vi "Add.vi"(1 "x":sgl, 2 "y":sgl, 4 "Adder":refnum<class "Adder.lvclass">) -> (6 "x+y":sgl)   [LabVIEW 2017, in "Adder.lvclass"]
uses:
  Adder.lvclass
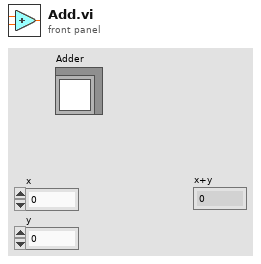
[diagram p1: front panel]
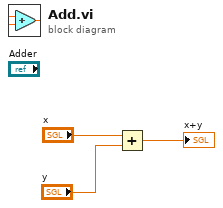
[diagram p0: block diagram]
diagram:
  n1 = Add(x="x", y="y") -> (x+y=→"x+y":sgl)
